vi "NiXnet ConvertTimestamp100nsTo1ns.vi"(6 "contextId":T1, 8 "error in":errorcluster, 9 "timeout (ms)":i32=-1, 10 "Request Data":T3, 11 "gRPC ID":T1) -> (0 "error out":errorcluster, 2 "Response Data":T2, 3 "gRPC ID out":T1)   [LabVIEW 2025, in "xnet-grpc_client.lvlib"]
uses:
  xnet-grpc_client.lvlib
  <vilib>/gRPC/LabVIEW gRPC Library/Shared/grpcId.ctl
  RPC Messages/nixnet_grpc_ConvertTimestamp100nsTo1nsRequest.ctl
  RPC Messages/nixnet_grpc_ConvertTimestamp100nsTo1nsResponse.ctl
  RPC Messages/nixnet_grpc_ConvertTimestamp100nsTo1nsResponse_Flat.ctl
  14035477-4c25-4107-8ed5-d0c4ef420ce5.vi
  <vilib>/gRPC/LabVIEW gRPC Library/Shared/TranslateGrpcError.vi
  <vilib>/gRPC/LabVIEW gRPC Library/Shared/Wait On Occurrence Wrapper.vi
  <vilib>/gRPC/LabVIEW gRPC Library/Shared/Wait On Occurence.vi
  <vilib>/gRPC/LabVIEW gRPC Library/Server API/Server/Get Server DLL Path.vi
  <vilib>/Utility/error.llb/Error Cluster From Error Code.vi
  <vilib>/Utility/config.llb/Open Config Data.vi
  <vilib>/Utility/config.llb/Write Key.vi
  <vilib>/Utility/config.llb/Write Key (Boolean).vi
  <vilib>/Utility/config.llb/Not A Config Data Refnum.vi
  <vilib>/Utility/config.llb/Read Key.vi
  <vilib>/Utility/config.llb/Read Key (Boolean).vi
  <vilib>/Utility/config.llb/Close Config Data.vi
  <vilib>/gRPC/LabVIEW gRPC Library/grpc-lvsupport-release.lvlib
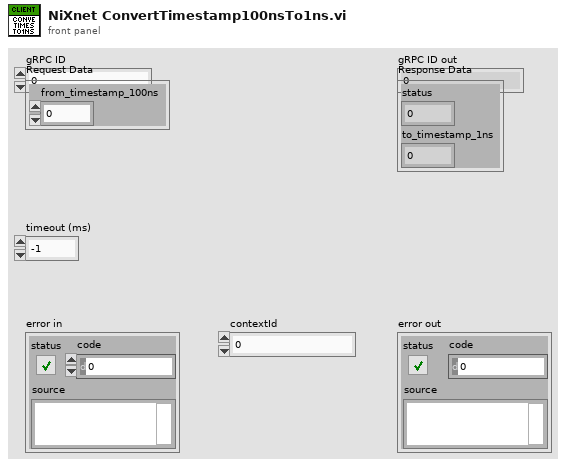
[diagram p1: front panel]
types:
  T1 = typedef "grpc-lvsupport-release.lvlib/grpcId.ctl" = u64
  T2 = typedef "xnet-grpc_client.lvlib/nixnet_grpc_ConvertTimestamp100nsTo1nsResponse.ctl" = cluster{"status":i32, "to_timestamp_1ns":u64}
  T3 = typedef "xnet-grpc_client.lvlib/nixnet_grpc_ConvertTimestamp100nsTo1nsRequest.ctl" = cluster{"from_timestamp_100ns":u64}
  T4 = typedef "xnet-grpc_client.lvlib/nixnet_grpc_ConvertTimestamp100nsTo1nsResponse_Flat.ctl" = cluster{"status":i32, "to_timestamp_1ns":u64}
  T5 = typedef "xnet-grpc_client.lvlib/nixnet_grpc_ConvertTimestamp100nsTo1nsRequest_Flat.ctl" = cluster{"from_timestamp_100ns":u64}
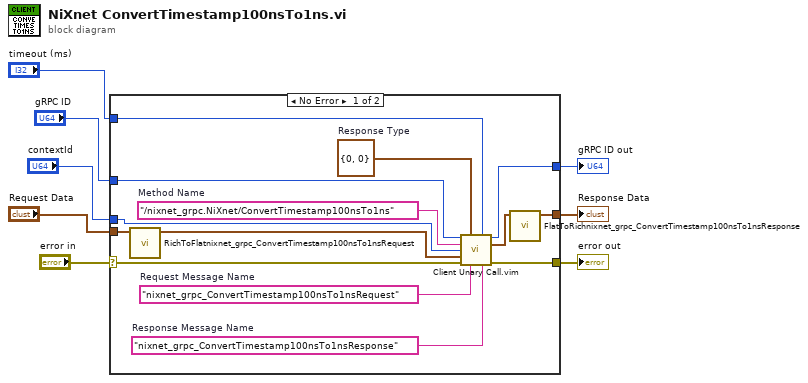
[diagram p0: block diagram]
diagram:
  n1 = case shown="No Error" "error in" {
    selector: "error in" -> [w18 w23]
    tunnel: [w17 w23] -> w7
    tunnel: "gRPC ID" -> [w16 w24]
    tunnel: [w15 w24] -> w5
    tunnel: "Request Data" -> [w12 _]
    tunnel: [w9 _] -> w3
    tunnel: "timeout (ms)" -> [w14 _]
    tunnel: "contextId" -> [w13 _]
    frame No Error {
      w19 = "nixnet_grpc_ConvertTimestamp100nsTo1nsResponse"  # Response Message Name
      w20 = "nixnet_grpc_ConvertTimestamp100nsTo1nsRequest"  # Request Message Name
      w21 = T4 {"status"=0, "to_timestamp_1ns"=0}  # Response Type
      w22 = "/nixnet_grpc.NiXnet/ConvertTimestamp100nsTo1ns"  # Method Name
      n2 = call "RichToFlatnixnet_grpc_ConvertTimestamp100nsTo1nsRequest.vi"("InputCluster"=w12) -> ("OutputCluster"=w11:T5)  [unwired: 10 in]
      n3 = call "Client Unary Call.vim"("ClientID in"=w16, "Response Type"=w21, "timeout (ms)"=w14, "Method Name"=w22, "contextId"=w13, "Request Data"=w11, "error in"=w18, "Request Message Name"=w20, "Response Message Name"=w19) -> ("ClientID out"=w15:u64, "Response Data"=w10:T4, "error out"=w17:errorcluster)  [unwired: 4 in]
      n4 = call "FlatToRichnixnet_grpc_ConvertTimestamp100nsTo1nsResponse.vi"("InputCluster"=w10) -> ("OutputCluster"=w9:T2)  [unwired: 10 in]
    }
    frame Error {
    }
  }
  "error out" <- w7
  "gRPC ID out" <- w5
  "Response Data" <- w3
